vi "Get Waveform.vi"(8 "error in (no error)":errorcluster, 11 "Logger in.lvclass":refnum<class "Logger.lvclass">) -> (0 "error out":errorcluster, 1 "Buffer Size":i32, 2 "Waveform Chart":waveform(dbl)[](graph), 3 "Logger out.lvclass":refnum<class "Logger.lvclass">)   [LabVIEW 2018, in "Logger.lvclass"]
uses:
  Logger.lvclass
  <vilib>/Waveform/WDTOps.llb/WDT Number of Waveform Samples DBL.vi
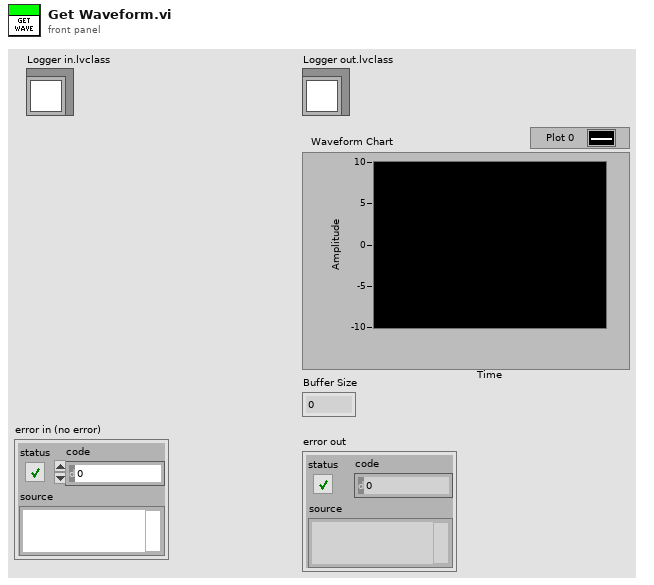
[diagram p1: front panel]
types:
  T1 = cluster{"Tag Units":string, "Tag Path":string, "Tag Reference":refnum<class "NI Skyline Tag.lvclass">}[]
  T2 = cluster{"Tag Units":string, "Tag Path":string, "Tag Reference":refnum<class "NI Skyline Tag.lvclass">}
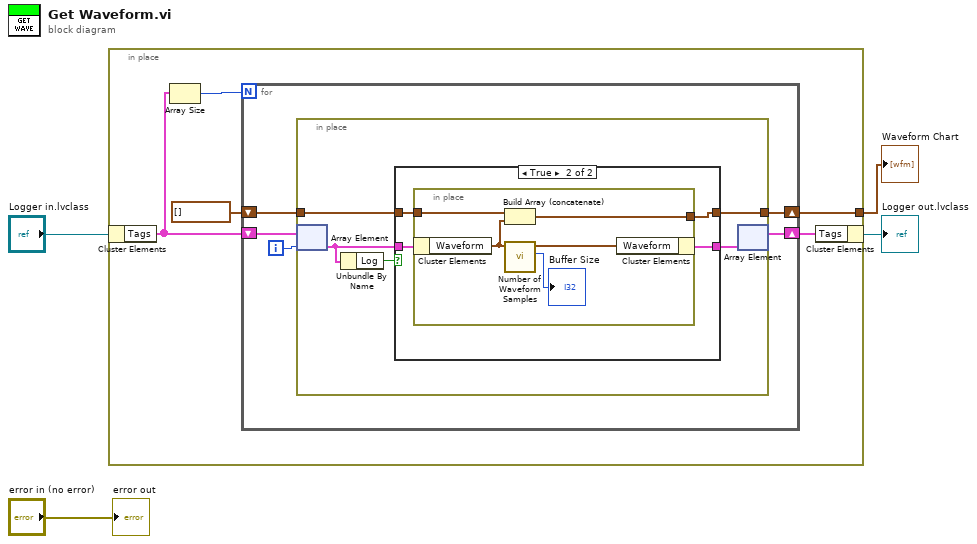
[diagram p0: block diagram]
diagram:
  n1 = in-place {
    in-place-border: [w5] -> w1
    n2 = in-place-cluster #1("Logger in.lvclass") -> ("Tags"=w7:T1)
    n3 = Array Size(array=w7) -> (size(s)=w8:i32)
    n4 = for {
      N: w8 -> [_]
      shift-right: [w12] -> w9
      shift-left: w7 -> [w14]
      shift-right: [w11] -> w5
      shift-left: waveform(dbl)[] [] -> [w10]
      i -> [w13]
      n5 = in-place {
        in-place-border: [w16] -> w11
        in-place-border: w10 -> [w15]
        n6 = in-place-array #2(w14, w13) -> (w18:T2)
        n7 = Unbundle By Name(w18) -> ("Log"=w17:bool)
        n8 = case shown="True" w17 {
          tunnel: w18 -> [w21 w25]
          tunnel: [w21 w24] -> w19
          tunnel: [w20 w23] -> w16
          tunnel: w15 -> [w20 w22]
          frame False {
          }
          frame True {
            n9 = in-place {
              in-place-border: [w30] -> w23
              in-place-border: w22 -> [w29]
              n10 = in-place-cluster #3(w25) -> ("Waveform"=w28:waveform(dbl))
              n11 = Build Array (concatenate)(w29, w28) -> (w30:waveform(dbl)[])
              n12 = call-poly <vilib>:"Number of Waveform Samples.vi"("waveform in"=w28) -> ("number of samples"=→"Buffer Size":i32, "waveform out"=w26:waveform(dbl))  [unwired: 8 in, 1 out]
              n13 = in-place-cluster #3("Waveform"=w26) -> (w24:T2)
            }
          }
        }
        n14 = in-place-array #2(w19) -> (w12:T1)  [unwired: 1 out]
      }
    }
    n15 = in-place-cluster #1("Tags"=w9) -> (→"Logger out.lvclass":refnum<class "Logger.lvclass">)
  }
  "Waveform Chart" <- w1
  "error out" <- "error in (no error)"
